vi "ELVIS III v1.0 Write DIO.vi"(8 "error in (no error)":errorcluster, 9 "bool Value List":bool[](array[boolean]), 10 "Channel List":T3, 11 "myRIO Ref In":T1) -> (0 "error out":errorcluster, 3 "myRIO Ref Out":T1)   [LabVIEW 2021]
uses:
  <vilib>/myRIO/Common/Instrument Driver Framework/myRIO v1.0/DIO/typedefs/DIO Channels List.ctl
  <vilib>/myRIO/Common/Instrument Driver Framework/myRIO v1.0/DIO/typedefs/DIO Channels Enum.ctl
  <vilib>/myRIO/Common/Instrument Driver Framework/Utilities/typedefs/myRIO v1.0 Reference.ctl
  <vilib>/myRIO/Common/Instrument Driver Framework/Utilities/typedefs/Generic FPGA Reference.ctl
  <vilib>/myRIO/Common/Instrument Driver Framework/ELVIS III v1.0/DIO/typedefs/ELVIS III DIO FPGA Reference.ctl
  <vilib>/myRIO/Common/Instrument Driver Framework/ELVIS III v1.0/DIO/typedefs/ELVIS III DIO Bank Enum.ctl
  <vilib>/rvi/errors/niLvFpgaAdjustHostInterfaceError.vi
  <vilib>/rvi/interface/nirviReadWriteControl/nirviReadWriteControl.xnode
  <vilib>/rvi/interface/Simulation/niFpgaSimulationCallBeginRW.vi
  NiFpgaLv.dll
panel:
  # "This VI writes boolean values to a user specified a list of DIO channels on the myRIO v1.0 hardware. The value is input as a boolean value. Please see Block Diagram for details."
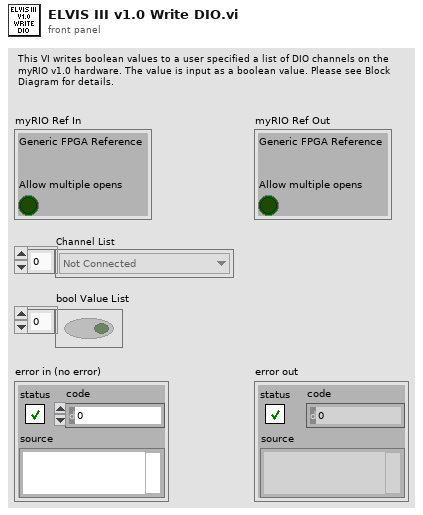
[diagram p1: front panel]
types:
  T1 = typedef "myRIO v1.0 Reference.ctl" = cluster{"Generic FPGA Reference":T2, "Allow multiple opens":bool}
  T2 = typedef "Generic FPGA Reference.ctl" = refnum<k20>
  T3 = typedef "DIO Channels List.ctl" = T4[]
  T4 = typedef "DIO Channels Enum.ctl" = enum16{"Not Connected", "C/DIO0", "C/DIO1", "C/DIO2", "C/DIO3", "C/DIO4", "C/DIO5", "C/DIO6", "C/DIO7", "A/DIO0", "A/DIO1", "A/DIO2", "A/DIO3", "A/DIO4", "A/DIO5", "A/DIO6", "A/DIO7", "A/DIO8", "A/DIO9", "A/DIO10", "A/DIO11", "A/DIO12", "A/DIO13", "A/DIO14", "A/DIO15", "A/DIO16", "A/DIO17", "A/DIO18", "A/DIO19", "B/DIO0", "B/DIO1", "B/DIO2", "B/DIO3", "B/DIO4", "B/DIO5", "B/DIO6", "B/DIO7", "B/DIO8", "B/DIO9", "B/DIO10", "B/DIO11", "B/DIO12", "B/DIO13", "B/DIO14", "B/DIO15", "B/DIO16", "B/DIO17", "B/DIO18", "B/DIO19", "LED0", "LED1", "LED2", "LED3", "Button0", "DIO/DIO0", "DIO/DIO1", "DIO/DIO2", "DIO/DIO3", "DIO/DIO4", "DIO/DIO5", "DIO/DIO6", "DIO/DIO7", "DIO/DIO8", "DIO/DIO9", "SPI/CS0", "SPI/CS1", "SPI/CS2", "SPI/CS3", "LED RADIO (Green)", "LED RADIO (Red)", "LED COMM (Green)", "LED COMM (Red)", "LED MODE (Green)", "LED MODE (Red)"}
  T5 = typedef "ELVIS III DIO Bank Enum.ctl" = enum32{"None", "A/DIO19:0", "B/DIO19:0", "LED3:0", "Button0"}
  T6 = typedef "ELVIS III DIO FPGA Reference.ctl" = refnum<k20>
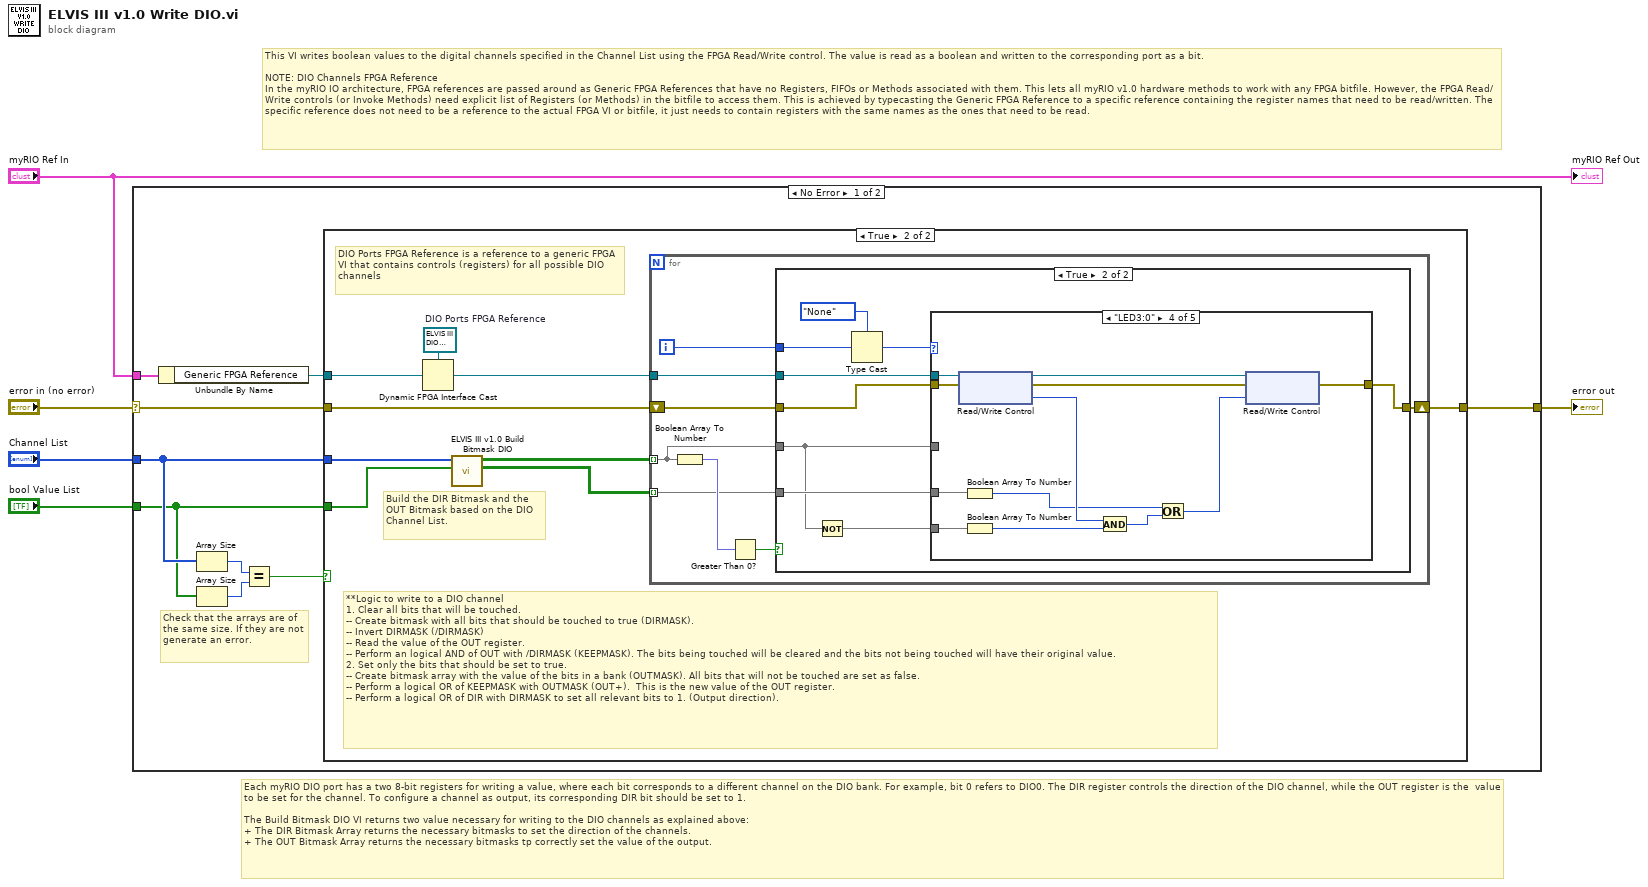
[diagram p0: block diagram]
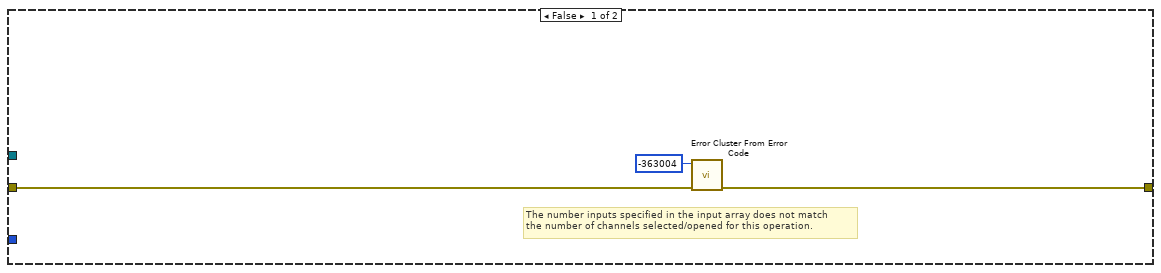
[diagram p2: hidden frame]
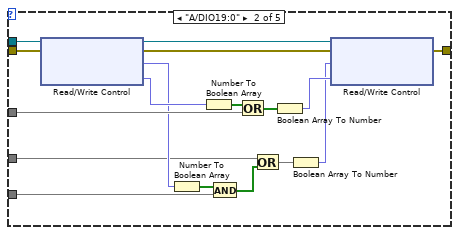
[diagram p5: hidden frame]
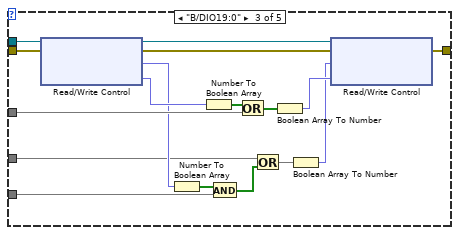
[diagram p6: hidden frame]
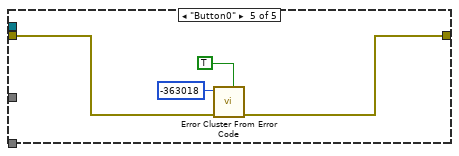
[diagram p7: hidden frame]
diagram:
  # "Each myRIO DIO port has a two 8-bit registers for writing a value, where each bit corresponds to a different channel on the DIO bank. For example, bit 0 refers to DIO0. The DIR register controls the direction of the DIO channel, while the OUT register is the  value to be set for the channel. To configure a channel as output, its corresponding DIR bit should be set to 1.\n\nThe Build Bitmask DIO VI returns two value necessary for writing to the DIO channels as explained above:\n+ The DIR Bitmask Array returns the necessary bitmasks to set the direction of the channels.\n+ The OUT Bitmask Array returns the necessary bitmasks tp correctly set the value of the output."
  # "This VI writes boolean values to the digital channels specified in the Channel List using the FPGA Read/Write control. The value is read as a boolean and written to the corresponding port as a bit. \n\nNOTE: DIO Channels FPGA Reference\nIn the myRIO IO architecture, FPGA references are passed around as Generic FPGA References that have no Registers, FIFOs or Methods associated with them. This lets all myRIO v1.0 hardware methods to work with any FPGA bitfile. However, the FPGA Read/Write controls (or Invoke Methods) need explicit list of Registers (or Methods) in the bitfile to access them. This is achieved by typecasting the Generic FPGA Reference to a specific reference containing the register names that need to be read/written. The specific reference does not need to be a reference to the actual FPGA VI or bitfile, it just needs to contain registers with the same names as the ones that need to be read."
  n1 = case shown="No Error" "error in (no error)" {
    selector: "error in (no error)" -> [w7 w96]
    tunnel: "myRIO Ref In" -> [w14 _]
    tunnel: [w13 w96] -> w4
    tunnel: "Channel List" -> [w10 _]
    tunnel: "bool Value List" -> [w9 _]
    frame No Error {
      # "Check that the arrays are of the same size. If they are not generate an error."
      n2 = Unbundle By Name(w14) -> ("Generic FPGA Reference"=w6:T2)
      n3 = Array Size(array=w10) -> (size(s)=w12:i32)
      n4 = Array Size(array=w9) -> (size(s)=w11:i32)
      n5 = Equal?(x=w12, y=w11) -> (x = y?=w8:bool)
      n6 = case shown="True" w8 {
        tunnel: w10 -> [_ w26]
        tunnel: w9 -> [_ w25]
        tunnel: w6 -> [_ w23]
        tunnel: w7 -> [w16 w21]
        tunnel: [w15 w20] -> w13
        frame False {
          # "The number inputs specified in the input array does not match\nthe number of channels selected/opened for this operation."
          n7 = call <vilib>:"Error Cluster From Error Code.vi"("error in (no error)"=w16, "error code (0)"=-363004) -> ("error out"=w15:errorcluster)  [unwired: 7 in]
        }
        frame True {
          w24 = T6 refnum  # DIO Ports FPGA Reference
          # "DIO Ports FPGA Reference is a reference to a generic FPGA VI that contains controls (registers) for all possible DIO channels"
          # "Build the DIR Bitmask and the OUT Bitmask based on the DIO Channel List."
          # "**Logic to write to a DIO channel\n1. Clear all bits that will be touched.\n-- Create bitmask with all bits that should be touched to true (DIRMASK).\n-- Invert DIRMASK (/DIRMASK)\n-- Read the value of the OUT register.\n-- Perform an logical AND of OUT with /DIRMASK (KEEPMASK). The bits being touched will be cleared and the bits not being touched will have their original value.\n2. Set only the bits that should be set to true.\n-- Create bitmask array with the value of the bits in a bank (OUTMASK). All bits that will not be touched are set as false.\n-- Perform a logical OR of KEEPMASK with OUTMASK (OUT+).  This is the new value of the OUT register.\n-- Perform a logical OR of DIR with DIRMASK to set all relevant bits to 1. (Output direction)."
          n8 = Dynamic FPGA Interface Cast(Session In=w24, Type=w23) -> (Session Out=w22:T6)
          n9 = call <vilib>:"ELVIS III v1.0 Build Bitmask DIO.vi"("bool Value List In"=w25, "Channel List"=w26) -> ("OUT Bitmask Array"=w18:bool[][], "DIR Bitmask Array"=w19:bool[][])  [unwired: 7 in, 1 out]
          n10 = for {
            tunnel: w22 -> [w34]
            tunnel: w19 -> [w27] mode=indexing
            shift-right: [w31] -> w20
            shift-left: w21 -> [w33]
            tunnel: w18 -> [w28] mode=indexing
            i -> [w32]
            n11 = Boolean Array To Number(Boolean array=w27) -> (number=w29:fxp<+,20,20>)
            n12 = Greater Than 0?(x=w29) -> (x > 0?=w30:bool)
            n13 = case shown="True" w30 {
              tunnel: w34 -> [_ w44]
              tunnel: w33 -> [w35 w43]
              tunnel: w32 -> [_ w41]
              tunnel: w28 -> [_ w39]
              tunnel: w27 -> [_ w36]
              tunnel: [w35 w37] -> w31
              frame False {
              }
              frame True {
                n14 = Not(x=w36) -> (.not. x?=w38:bool[])
                n15 = Type Cast(type=ELVIS_III_DIO_Bank_Enum."None" ("DIO Bank Enum"), x=w41) -> (*(type *) &x=w40:T5)
                n16 = case shown="\"LED3:0\"" w40 {
                  tunnel: w44 -> [_ w62 w79 w85 _]
                  tunnel: w43 -> [w45 w46 w63 w84 w95]
                  tunnel: w36 -> [_ w59 w76 _ _]
                  tunnel: w39 -> [_ w52 w69 w83 _]
                  tunnel: w38 -> [_ w55 w72 w81 _]
                  tunnel: [w45 w48 w65 w86 w94] -> w37
                  frame "None", Default {
                  }
                  frame "A/DIO19:0" {
                    n17 = xnode "Read/Write Control"("FPGA VI Reference In"=w62, "error in"=w46) -> ("FPGA VI Reference Out"=w61:T6, "error out"=w47:errorcluster, "DIO.A_19:0.OUT"=w54:fxp<+,20,20>, "DIO.A_19:0.DIR"=w58:fxp<+,20,20>)
                    n18 = Number To Boolean Array(number=w54) -> (Boolean array=w53:bool[])
                    n19 = Number To Boolean Array(number=w58) -> (Boolean array=w60:bool[])
                    n20 = And(x=w53, y=w55) -> (x .and. y?=w51:bool[])
                    n21 = Or(x=w60, y=w59) -> (x .or. y?=w57:bool[])
                    n22 = Or(x=w52, y=w51) -> (x .or. y?=w50:bool[])
                    n23 = Boolean Array To Number(Boolean array=w57) -> (number=w56:fxp<+,20,20>)
                    n24 = Boolean Array To Number(Boolean array=w50) -> (number=w49:fxp<+,20,20>)
                    n25 = xnode "Read/Write Control"("FPGA VI Reference In"=w61, "error in"=w47, "DIO.A_19:0.OUT"=w49, "DIO.A_19:0.DIR"=w56) -> ("error out"=w48:errorcluster)  [unwired: 1 out]
                  }
                  frame "B/DIO19:0" {
                    n26 = xnode "Read/Write Control"("FPGA VI Reference In"=w79, "error in"=w63) -> ("FPGA VI Reference Out"=w78:T6, "error out"=w64:errorcluster, "DIO.B_19:0.OUT"=w71:fxp<+,20,20>, "DIO.B_19:0.DIR"=w75:fxp<+,20,20>)
                    n27 = Number To Boolean Array(number=w71) -> (Boolean array=w70:bool[])
                    n28 = Number To Boolean Array(number=w75) -> (Boolean array=w77:bool[])
                    n29 = And(x=w70, y=w72) -> (x .and. y?=w68:bool[])
                    n30 = Or(x=w77, y=w76) -> (x .or. y?=w74:bool[])
                    n31 = Or(x=w69, y=w68) -> (x .or. y?=w67:bool[])
                    n32 = Boolean Array To Number(Boolean array=w74) -> (number=w73:fxp<+,20,20>)
                    n33 = Boolean Array To Number(Boolean array=w67) -> (number=w66:fxp<+,20,20>)
                    n34 = xnode "Read/Write Control"("FPGA VI Reference In"=w78, "error in"=w64, "DIO.B_19:0.OUT"=w66, "DIO.B_19:0.DIR"=w73) -> ("error out"=w65:errorcluster)  [unwired: 1 out]
                  }
                  frame "LED3:0" {
                    n35 = xnode "Read/Write Control"("FPGA VI Reference In"=w85, "error in"=w84) -> ("FPGA VI Reference Out"=w88:T6, "error out"=w87:errorcluster, "DO.LED3:0"=w91:u8)
                    n36 = Boolean Array To Number(Boolean array=w83) -> (number=w82:u8)
                    n37 = Boolean Array To Number(Boolean array=w81) -> (number=w80:u8)
                    n38 = And(x=w91, y=w80) -> (x .and. y?=w90:u8)
                    n39 = Or(x=w82, y=w90) -> (x .or. y?=w89:u8)
                    n40 = xnode "Read/Write Control"("FPGA VI Reference In"=w88, "error in"=w87, "DO.LED3:0"=w89) -> ("error out"=w86:errorcluster)  [unwired: 1 out]
                  }
                  frame "Button0" {
                    n41 = call <vilib>:"Error Cluster From Error Code.vi"("is warning? (False)"=TRUE, "error in (no error)"=w95, "error code (0)"=-363018) -> ("error out"=w94:errorcluster)  [unwired: 6 in]
                  }
                }
              }
            }
          }
        }
      }
    }
    frame Error {
    }
  }
  "error out" <- w4
  "myRIO Ref Out" <- "myRIO Ref In"
